vi "Initialize DMA.vi"(7 "Number of Channels":u8, 8 "error in (no error)":errorcluster, 9 "dt":dbl, 10 "DMA Ref":T1, 11 "Multiple Waveforms Write (DBL) in":refnum<class "Multiple Waveforms Write (DBL).lvclass">) -> (0 "error out":errorcluster, 2 "DMA Ref":T1, 3 "Multiple Waveforms Write (DBL) out":refnum<class "Multiple Waveforms Write (DBL).lvclass">)   [LabVIEW 2016, in "FPGA Addon Engine.lvlib"]
uses:
  FPGA Addon Engine.lvlib
  Types/DMA Input Ref.ctl
  <vilib>/NI Veristand/Custom Device Waveform API/Multiple Waveforms Write (DBL)/Multiple Waveforms Write (DBL).lvclass
  C:/Program Files (x86)/National Instruments/LabVIEW 2016/vi.lib/NI Veristand/Custom Device Waveform API/Waveform Session.lvclass
  <vilib>/NI Veristand/Custom Device Waveform API/Waveform Session.lvclass/Waveform Session.ctl
  <vilib>/NI Veristand/Custom Device Waveform API/Multiple Waveforms Write (DBL)/Multiple Waveforms Write (DBL).lvclass/Multiple Waveforms Write (DBL).ctl
  <vilib>/NI Veristand/Custom Device Waveform API/Internal Comm Classes/WPL Comm/WPL Comm.lvclass/WPL Comm.ctl
  <vilib>/NI Veristand/Custom Device Waveform API/Multiple Waveforms Write (DBL)/NI VeriStand - Start Multiple Waveforms (DBL).vi
  <vilib>/NI Veristand/Custom Device Waveform API/Internal Comm Classes/WPL Comm/WPL_start dbl waveform.vi
  <vilib>/NI Veristand/Custom Device Waveform API/Read Sample offset DVR.vi
  <vilib>/NI Veristand/Custom Device Waveform API/Check Opened.vi
  <vilib>/NI Veristand/Custom Device Waveform API/Internal Comm Classes/WPL Comm/Set t0 on Variant.vi
  <vilib>/NI Veristand/Custom Device Waveform API/Internal Comm Classes/WPL Comm/Send WPL Command.vi
  <vilib>/NI Veristand/Custom Device Waveform API/Internal Comm Classes/WPL Comm/Convert Q Error to Shutdown Error.vi
  <vilib>/NI Veristand/Custom Device Waveform API/Internal Comm Classes/WPL Comm/WPL Comm (2D DBL)/WPL Comm (2D DBL).lvclass
  C:/Program Files (x86)/National Instruments/LabVIEW 2016/vi.lib/NI Veristand/Custom Device Waveform API/Internal Comm Classes/WPL Comm/WPL Comm.lvclass
  <vilib>/Utility/error.llb/Error Cluster From Error Code.vi
  <vilib>/rvi/errors/niLvFpgaAdjustHostInterfaceError.vi
  <vilib>/rvi/interface/nirviMethod/nirviMethod.xnode
  <vilib>/NI VeriStand/Custom Device Waveform API/NI_VS Custom Device Waveform API.lvlib
  <vilib>/FPGAPlugInAG/Dynamic/niLvFpga_ReadFifo_Dynamic.vi
  <vilib>/rvi/errors/niLvFpgaMergeErrorWithErrorCode.vi
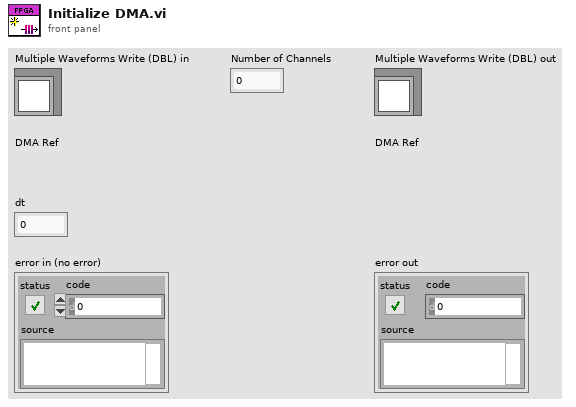
[diagram p1: front panel]
types:
  T1 = typedef "FPGA Addon Engine.lvlib/DMA Input Ref.ctl" = refnum<k20>
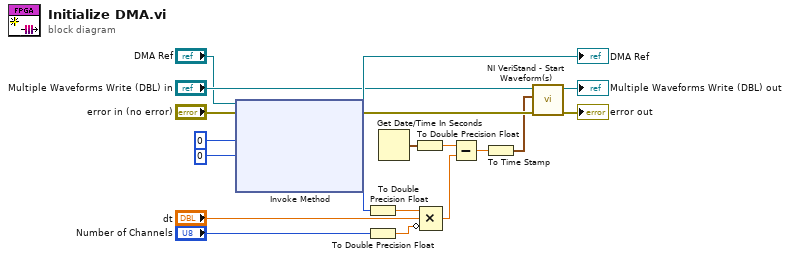
[diagram p0: block diagram]
diagram:
  n1 = xnode "Invoke Method"("FPGA VI Reference In"="DMA Ref", "error in"="error in (no error)", "Number of Elements"=u32 0, "Timeout (ms)"=0) -> ("FPGA VI Reference Out"=→"DMA Ref":T1, "error out"=w14:errorcluster, "Elements Remaining"=w8:u32)  [unwired: 1 out]
  n2 = To Double Precision Float(number=w8) -> (double precision float=w9:dbl)
  n3 = To Double Precision Float(number="Number of Channels") -> (double precision float=w7:dbl)
  n4 = Get Date/Time In Seconds() -> (seconds since 1Jan1904=w6:timestamp)
  n5 = To Double Precision Float(number=w6) -> (double precision float=w4:dbl)
  n6 = Compound Arithmetic op=MULTIPLY(w9, "dt", invert w7) -> (w5:dbl)
  n7 = Subtract(x=w4, y=w5) -> (x-y=w10:dbl)
  n8 = To Time Stamp(1:w10) -> (0:w13:timestamp)
  n9 = call-poly <vilib>:"NI VeriStand - Start Waveform(s).vi"("error in (no error)"=w14, "t0"=w13, "Multiple Waveforms Write Session (DBL) in"="Multiple Waveforms Write (DBL) in") -> ("error out"=→"error out":errorcluster, "Multiple Waveforms Write Session (DBL) out"=→"Multiple Waveforms Write (DBL) out":refnum<class "Multiple Waveforms Write (DBL).lvclass">)  [unwired: 7 in]
